vi "load_xml.vi"(8 "error in":errorcluster, 10 "child node in":refnum<k20>, 11 "Hamamatsu_C9100-13.lvclass (in)":refnum<class "Hamamatsu_C9100-13.lvclass">) -> (0 "error out":errorcluster, 2 "child node out":refnum<k20>, 3 "Hamamatsu_C9100-13.lvclass":refnum<class "Hamamatsu_C9100-13.lvclass">)   [LabVIEW 2013, in "Hamamatsu_C9100-13.lvclass"]
doc: "Loads Hamamatsu C9100-13 camera settings from xml. Expected format:\n\n<Enable>%b</Enable>\n<AnalogGain>%u</AnalogGain>\n<FrameGrabberAcquisitionRegion columns=\"left, top, right, bottom\">%u %u %u %u</FrameGrabberAcquisitionRegion>\n<ExposureTime>%f</ExposureTime>\n<EMGain>%u</EMGain>\n<TriggerPolarity>%s</TriggerPolarity>\n<ExternalTriggerMode>%s</ExternalTriggerMode>\n<ScanSpeed>%s</ScanSpeed>\n<ExternalTriggerSource>%s</ExternalTriggerSource>\n<ScanMode>%s</ScanMode>\n<SuperPixelBinning>%s</SuperPixelBinning>\n<CameraSubArrayAcquisitionRegion columns=\"left, top, width, height\">%u %u %u %u</CameraSubArrayAcquisitionRegion>\n<NumberOfImageBuffers>%u</NumberOfImageBuffers>\n<RegionsOfInterest columns=\"Left, Top, Right Bottom\">\n%s</RegionsOfInterest>\n<BackgroundRegions columns=\"Left, Top, Right Bottom\">\n%s</BackgroundRegions>\n<ShotsPerMeasurement>%u</ShotsPerMeasurement>\n<PhotoelectronScaling>%f</PhotoelectronScaling>\n\nMTL 2013 Jan 1"
uses:
  Hamamatsu_C9100-13.lvclass
  Hamamatsu_C9100-13.lvclass/Hamamatsu_C9100-13.ctl
  Experiment/Globals.vi
  <vilib>/xml/Close Reference(Node).vi
  <resource>/objmgr/DOMUserDefRef.rc
  <vilib>/xml/NI_XML.lvlib
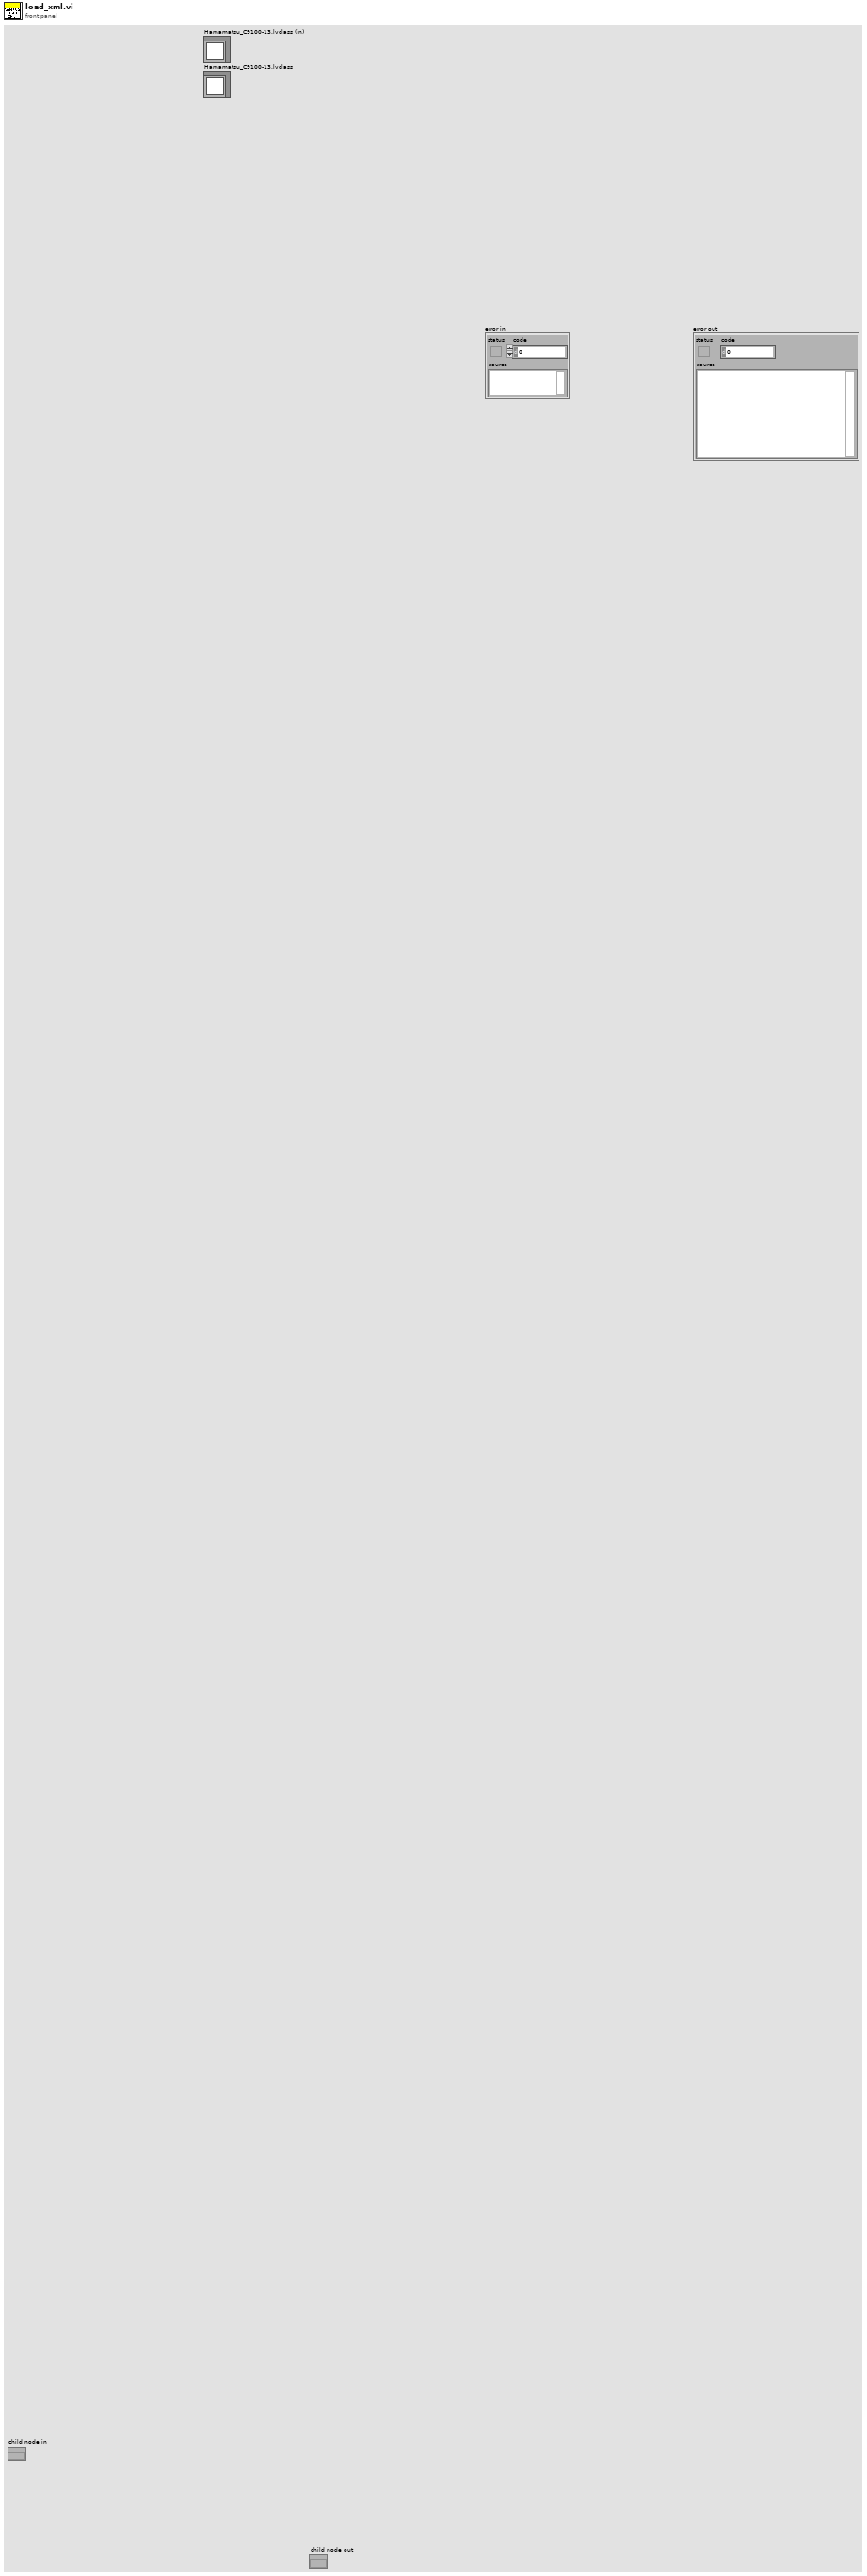
[diagram p1: front panel]
types:
  T1 = typedef "Hamamatsu_C9100-13.lvclass/camera_setup.ctl" = cluster{"Analog Gain (0-5)":u8, "Exposure Time":dbl, "EM Gain (0-255)":u8, "Trigger Polarity":string, "External Trigger Mode":string, "Scan Speed":string, "External Trigger Source":string, "Scan Mode":string, "Super Pixel Binning\n(if enabled in Scan Mode)":string, "Camera Sub-array acquisition region\n(if enabled in scan mode)":cluster{"Left":u16, "Top":u16, "Width":u16, "Height":u16}, "Use camera?":bool, "# image buffers":i32, "shots per measurement":i32, "Force images to U16":bool, "Low Light Sensitivity":string, "cooling":string, "fan":string, "Frame Grabber acquisition region":cluster{"Left":i32, "Top":i32, "Right":i32, "Bottom":i32}}
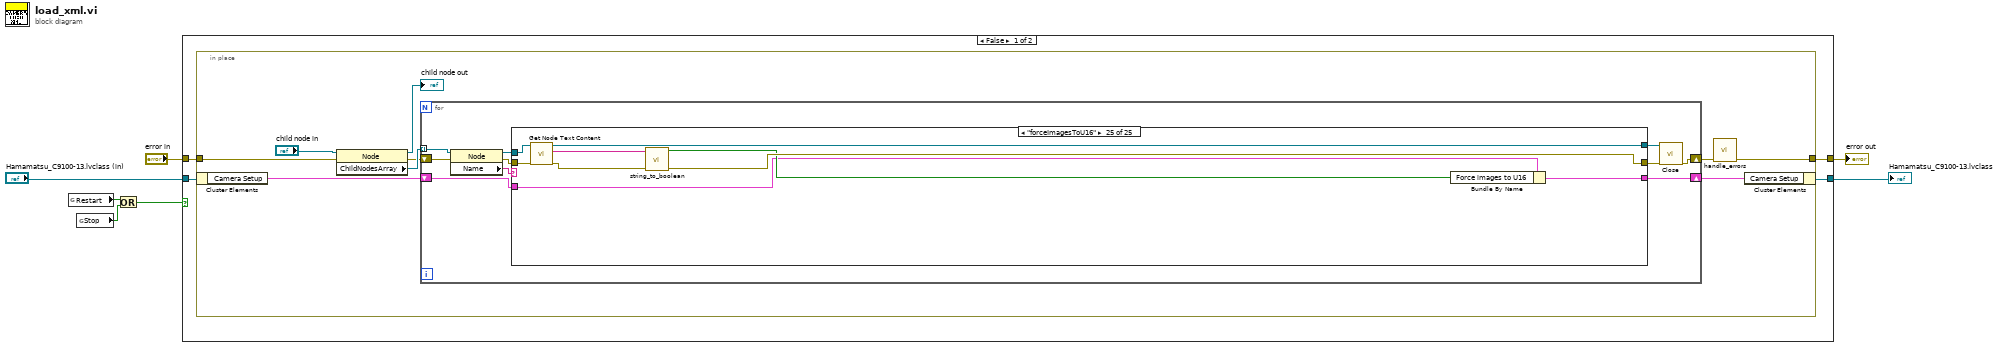
[diagram p0: block diagram]
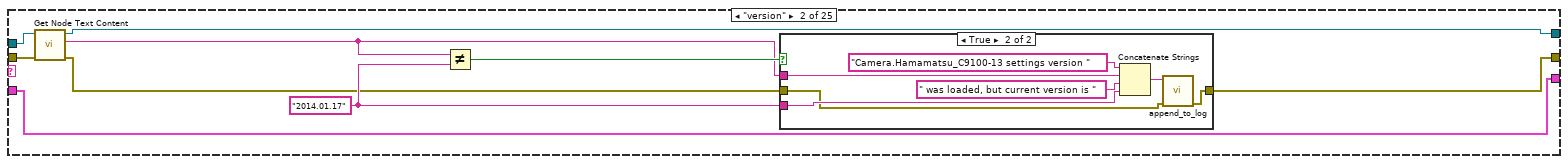
[diagram p3: hidden frame]
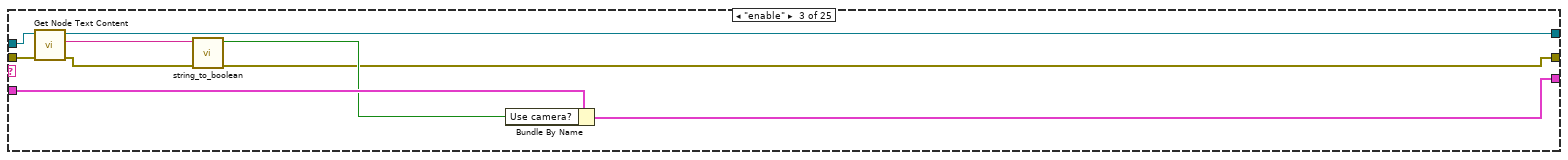
[diagram p5: hidden frame]
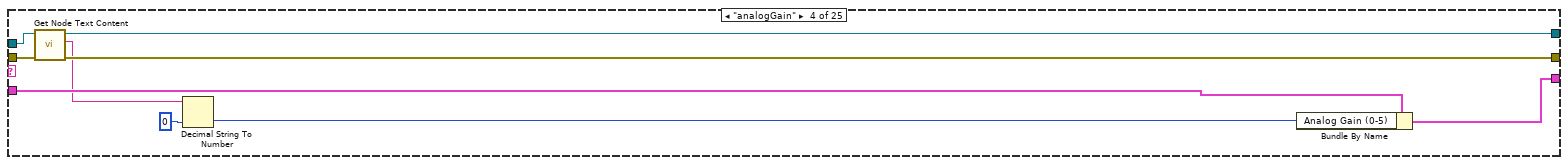
[diagram p6: hidden frame]
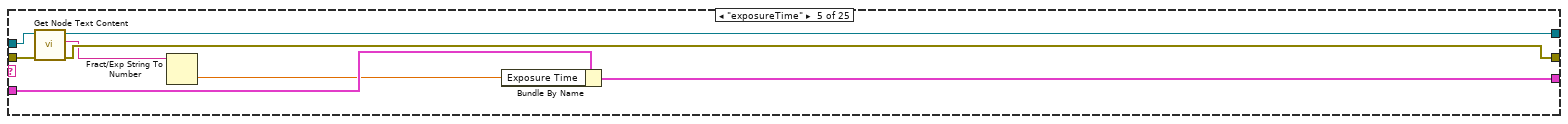
[diagram p7: hidden frame]
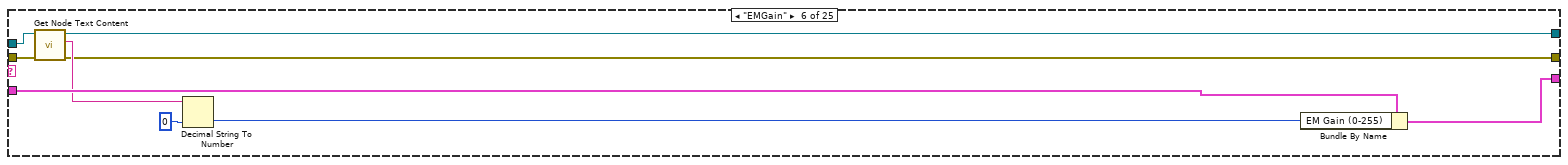
[diagram p8: hidden frame]
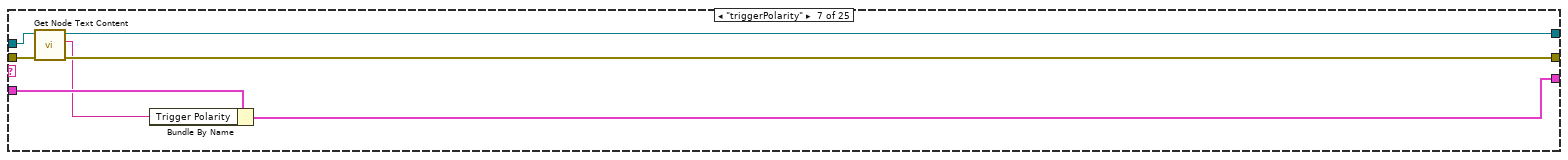
[diagram p9: hidden frame]
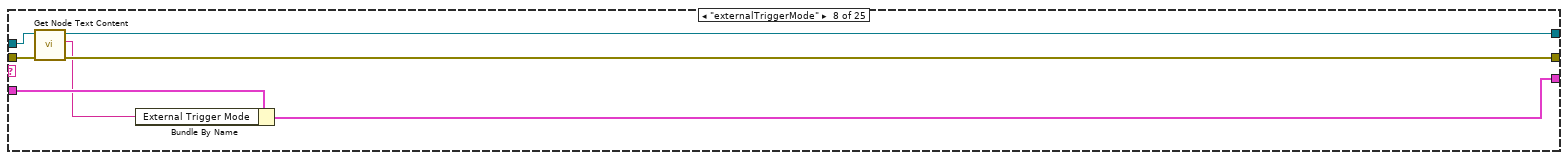
[diagram p10: hidden frame]
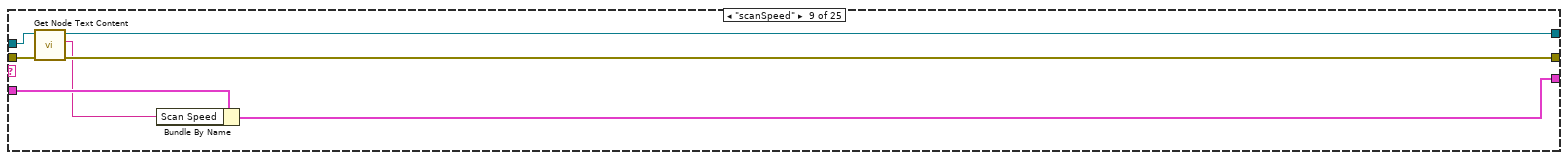
[diagram p11: hidden frame]
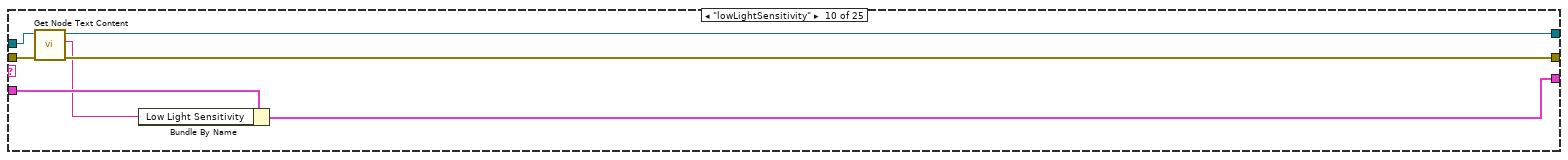
[diagram p12: hidden frame]
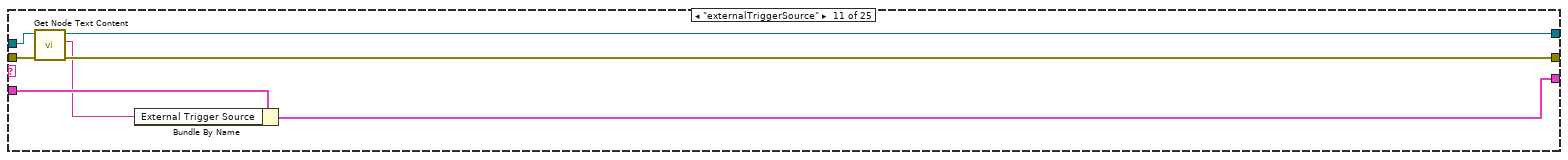
[diagram p13: hidden frame]
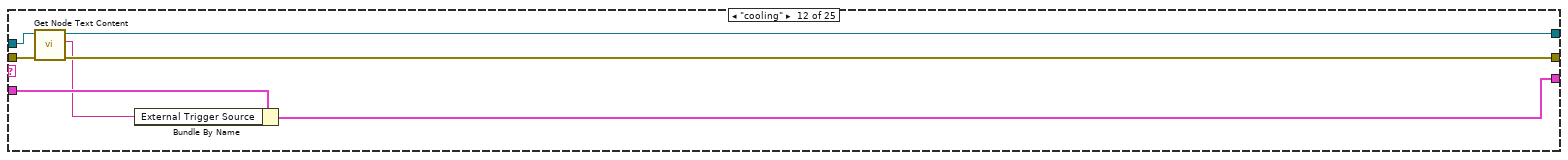
[diagram p14: hidden frame]
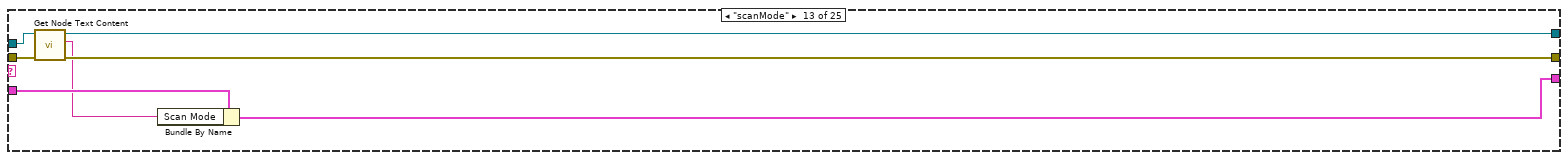
[diagram p15: hidden frame]
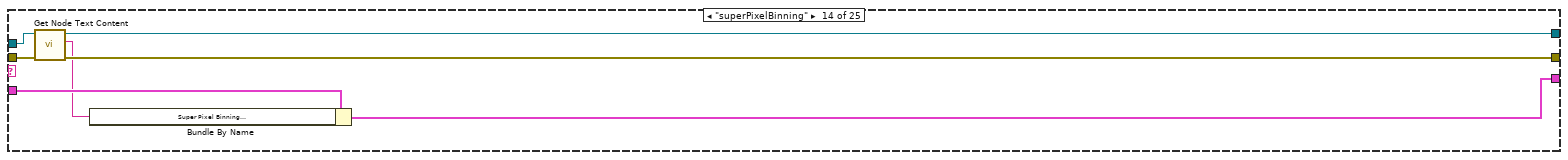
[diagram p16: hidden frame]
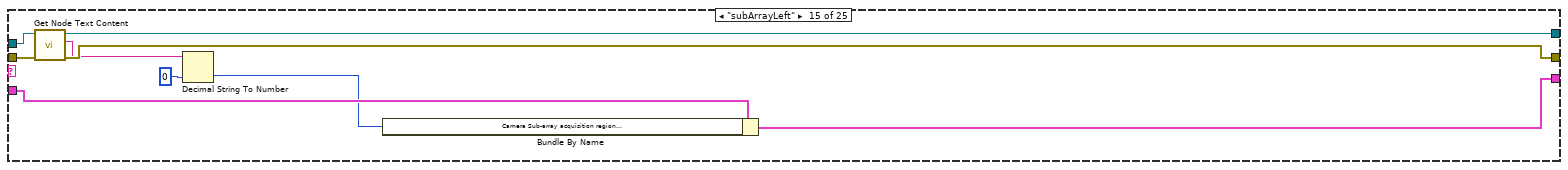
[diagram p17: hidden frame]
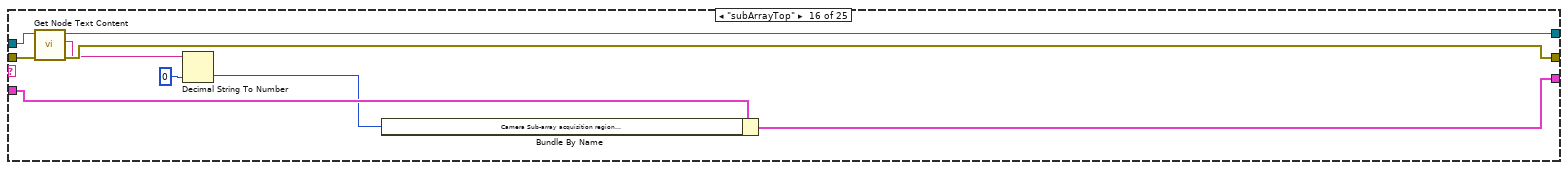
[diagram p18: hidden frame]
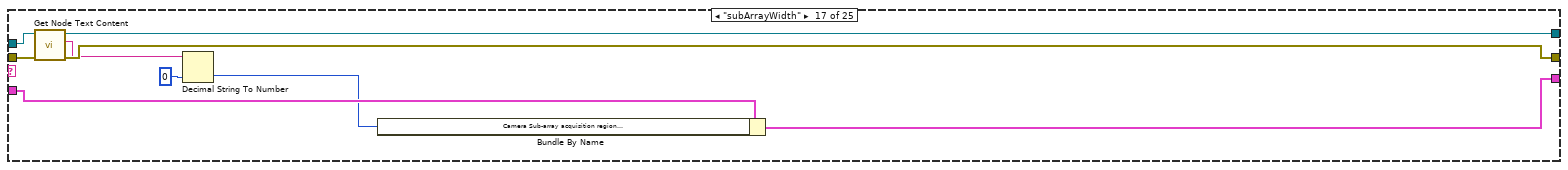
[diagram p19: hidden frame]
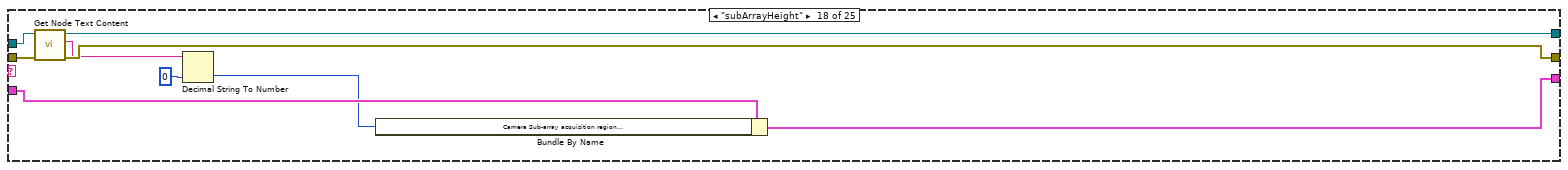
[diagram p20: hidden frame]
diagram:
  n1 = global read "Globals.vi" "Restart"() -> (w6:bool)
  n2 = global read "Globals.vi" "Stop"() -> (w5:bool)
  n3 = Or(x=w6, y=w5) -> (x .or. y?=w4:bool)
  n4 = case shown="False" w4 {
    tunnel: [w11 w242] -> w7
    tunnel: "error in" -> [w10 w242]
    tunnel: "Hamamatsu_C9100-13.lvclass (in)" -> [w9 w241]
    tunnel: [w8 w241] -> w1
    frame False {
      n5 = in-place {
        in-place-border: [w15] -> w11
        in-place-border: w10 -> [w14]
        n6 = in-place-cluster #1(w9) -> ("Camera Setup"=w12:T1)
        n7 = property class="Node"(reference="child node in", error in=w14) -> (reference out=→"child node out":refnum<k20>, error out=w18:errorcluster, "ChildNodesArray"=w20:refnum<k20>[])
        n8 = for {
          tunnel: w20 -> [w21] mode=indexing
          shift-right: [w27] -> w13
          shift-left: w12 -> [w28]
          shift-right: [w24] -> w16
          shift-left: w18 -> [w22]
          n9 = property class="Node"(reference=w21, error in=w22) -> (reference out=w29:refnum<k20>, error out=w25:errorcluster, "Name"=w30:string)
          n10 = case shown="\"forceImagesToU16\"" w30 {
            tunnel: w29 -> [w32 w37 w58 w65 w73 w84 w89 w96 w103 w110 w117 w124 w131 w138 w149 w158 w167 w176 w185 w194 w203 w212 w221 w230 w239]
            tunnel: w28 -> [w33 w36 w56 w68 w76 w82 w92 w99 w106 w113 w120 w127 w134 w141 w146 w155 w164 w173 w182 w191 w200 w209 w219 w228 w232]
            tunnel: [w33 w36 w55 w67 w75 w81 w91 w98 w105 w112 w119 w126 w133 w140 w142 w151 w160 w169 w178 w187 w196 w205 w218 w227 w237] -> w27
            tunnel: [w32 w35 w59 w66 w74 w85 w90 w97 w104 w111 w118 w125 w132 w139 w147 w156 w165 w174 w183 w192 w201 w210 w222 w231 w240] -> w26
            tunnel: w25 -> [w31 w38 w57 w64 w72 w83 w88 w95 w102 w109 w116 w123 w130 w137 w150 w159 w168 w177 w186 w195 w204 w213 w220 w229 w238]
            tunnel: [w31 w34 w51 w63 w71 w79 w87 w94 w101 w108 w115 w122 w129 w136 w148 w157 w166 w175 w184 w193 w202 w211 w216 w225 w235] -> w23
            frame "None", Default {
            }
            frame "version" {
              w40 = "2014.01.17" ("y")
              n11 = call <vilib>:"Get Node Text Content.vi"("error in (no error)"=w38, "node in"=w37) -> ("error out"=w39:errorcluster, "node text"=w41:string, "node out"=w35:refnum<k20>)  [unwired: 7 in]
              n12 = Not Equal?(x=w41, y=w40) -> (x != y?=w42:bool)
              n13 = case shown="True" w42 {
                tunnel: w41 -> [_ w49]
                tunnel: w40 -> [_ w47]
                tunnel: w39 -> [w43 w45]
                tunnel: [w43 w44] -> w34
                frame False {
                }
                frame True {
                  n14 = Concatenate Strings("Camera.Hamamatsu_C9100-13 settings version " ("string"), w49, " was loaded, but current version is " ("string"), w47) -> (w46:string)
                  n15 = call "append_to_log.vi"("error in"=w45, "string"=w46) -> ("error out"=w44:errorcluster)  [unwired: 9 in]
                }
              }
            }
            frame "enable" {
              n16 = call <vilib>:"Get Node Text Content.vi"("error in (no error)"=w57, "node in"=w58) -> ("error out"=w53:errorcluster, "node text"=w54:string, "node out"=w59:refnum<k20>)  [unwired: 7 in]
              n17 = call "string_to_boolean.vi"("error in"=w53, "string"=w54) -> ("error out"=w51:errorcluster, "boolean"=w52:bool)  [unwired: 8 in]
              n18 = Bundle By Name(cluster=w56, "Use camera?"=w52) -> (w55:T1)
            }
            frame "analogGain" {
              n19 = call <vilib>:"Get Node Text Content.vi"("error in (no error)"=w64, "node in"=w65) -> ("error out"=w63:errorcluster, "node text"=w62:string, "node out"=w66:refnum<k20>)  [unwired: 7 in]
              n20 = Decimal String To Number(string=w62, default (0L)=u8 0 ("Analog Gain (0-5)")) -> (number=w60:u8)  [unwired: 1 in, 1 out]
              n21 = Bundle By Name(cluster=w68, "Analog Gain (0-5)"=w60) -> (w67:T1)
            }
            frame "exposureTime" {
              n22 = call <vilib>:"Get Node Text Content.vi"("error in (no error)"=w72, "node in"=w73) -> ("error out"=w71:errorcluster, "node text"=w70:string, "node out"=w74:refnum<k20>)  [unwired: 7 in]
              n23 = Fract/Exp String To Number(string=w70) -> (number=w69:dbl)  [unwired: 3 in, 1 out]
              n24 = Bundle By Name(cluster=w76, "Exposure Time"=w69) -> (w75:T1)
            }
            frame "EMGain" {
              n25 = call <vilib>:"Get Node Text Content.vi"("error in (no error)"=w83, "node in"=w84) -> ("error out"=w79:errorcluster, "node text"=w80:string, "node out"=w85:refnum<k20>)  [unwired: 7 in]
              n26 = Decimal String To Number(string=w80, default (0L)=u8 0 ("EM Gain (0-255)")) -> (number=w77:u8)  [unwired: 1 in, 1 out]
              n27 = Bundle By Name(cluster=w82, "EM Gain (0-255)"=w77) -> (w81:T1)
            }
            frame "triggerPolarity" {
              n28 = call <vilib>:"Get Node Text Content.vi"("error in (no error)"=w88, "node in"=w89) -> ("error out"=w87:errorcluster, "node text"=w86:string, "node out"=w90:refnum<k20>)  [unwired: 7 in]
              n29 = Bundle By Name(cluster=w92, "Trigger Polarity"=w86) -> (w91:T1)
            }
            frame "externalTriggerMode" {
              n30 = call <vilib>:"Get Node Text Content.vi"("error in (no error)"=w95, "node in"=w96) -> ("error out"=w94:errorcluster, "node text"=w93:string, "node out"=w97:refnum<k20>)  [unwired: 7 in]
              n31 = Bundle By Name(cluster=w99, "External Trigger Mode"=w93) -> (w98:T1)
            }
            frame "scanSpeed" {
              n32 = call <vilib>:"Get Node Text Content.vi"("error in (no error)"=w102, "node in"=w103) -> ("error out"=w101:errorcluster, "node text"=w100:string, "node out"=w104:refnum<k20>)  [unwired: 7 in]
              n33 = Bundle By Name(cluster=w106, "Scan Speed"=w100) -> (w105:T1)
            }
            frame "lowLightSensitivity" {
              n34 = call <vilib>:"Get Node Text Content.vi"("error in (no error)"=w109, "node in"=w110) -> ("error out"=w108:errorcluster, "node text"=w107:string, "node out"=w111:refnum<k20>)  [unwired: 7 in]
              n35 = Bundle By Name(cluster=w113, "Low Light Sensitivity"=w107) -> (w112:T1)
            }
            frame "externalTriggerSource" {
              n36 = call <vilib>:"Get Node Text Content.vi"("error in (no error)"=w116, "node in"=w117) -> ("error out"=w115:errorcluster, "node text"=w114:string, "node out"=w118:refnum<k20>)  [unwired: 7 in]
              n37 = Bundle By Name(cluster=w120, "External Trigger Source"=w114) -> (w119:T1)
            }
            frame "cooling" {
              n38 = call <vilib>:"Get Node Text Content.vi"("error in (no error)"=w123, "node in"=w124) -> ("error out"=w122:errorcluster, "node text"=w121:string, "node out"=w125:refnum<k20>)  [unwired: 7 in]
              n39 = Bundle By Name(cluster=w127, "External Trigger Source"=w121) -> (w126:T1)
            }
            frame "scanMode" {
              n40 = call <vilib>:"Get Node Text Content.vi"("error in (no error)"=w130, "node in"=w131) -> ("error out"=w129:errorcluster, "node text"=w128:string, "node out"=w132:refnum<k20>)  [unwired: 7 in]
              n41 = Bundle By Name(cluster=w134, "Scan Mode"=w128) -> (w133:T1)
            }
            frame "superPixelBinning" {
              n42 = call <vilib>:"Get Node Text Content.vi"("error in (no error)"=w137, "node in"=w138) -> ("error out"=w136:errorcluster, "node text"=w135:string, "node out"=w139:refnum<k20>)  [unwired: 7 in]
              n43 = Bundle By Name(cluster=w141, "Super Pixel Binning\n(if enabled in Scan Mode)"=w135) -> (w140:T1)
            }
            frame "subArrayLeft" {
              n44 = call <vilib>:"Get Node Text Content.vi"("error in (no error)"=w150, "node in"=w149) -> ("error out"=w148:errorcluster, "node text"=w144:string, "node out"=w147:refnum<k20>)  [unwired: 7 in]
              n45 = Decimal String To Number(string=w144, default (0L)=u16 0 ("EM Gain (0-255)")) -> (number=w143:u16)  [unwired: 1 in, 1 out]
              n46 = Bundle By Name(cluster=w146, "Camera Sub-array acquisition region\n(if enabled in scan mode).Left"=w143) -> (w142:T1)
            }
            frame "subArrayTop" {
              n47 = call <vilib>:"Get Node Text Content.vi"("error in (no error)"=w159, "node in"=w158) -> ("error out"=w157:errorcluster, "node text"=w153:string, "node out"=w156:refnum<k20>)  [unwired: 7 in]
              n48 = Decimal String To Number(string=w153, default (0L)=u16 0 ("EM Gain (0-255)")) -> (number=w152:u16)  [unwired: 1 in, 1 out]
              n49 = Bundle By Name(cluster=w155, "Camera Sub-array acquisition region\n(if enabled in scan mode).Top"=w152) -> (w151:T1)
            }
            frame "subArrayWidth" {
              n50 = call <vilib>:"Get Node Text Content.vi"("error in (no error)"=w168, "node in"=w167) -> ("error out"=w166:errorcluster, "node text"=w162:string, "node out"=w165:refnum<k20>)  [unwired: 7 in]
              n51 = Decimal String To Number(string=w162, default (0L)=u16 0 ("EM Gain (0-255)")) -> (number=w161:u16)  [unwired: 1 in, 1 out]
              n52 = Bundle By Name(cluster=w164, "Camera Sub-array acquisition region\n(if enabled in scan mode).Width"=w161) -> (w160:T1)
            }
            frame "subArrayHeight" {
              n53 = call <vilib>:"Get Node Text Content.vi"("error in (no error)"=w177, "node in"=w176) -> ("error out"=w175:errorcluster, "node text"=w171:string, "node out"=w174:refnum<k20>)  [unwired: 7 in]
              n54 = Decimal String To Number(string=w171, default (0L)=u16 0 ("EM Gain (0-255)")) -> (number=w170:u16)  [unwired: 1 in, 1 out]
              n55 = Bundle By Name(cluster=w173, "Camera Sub-array acquisition region\n(if enabled in scan mode).Height"=w170) -> (w169:T1)
            }
            frame "frameGrabberAcquisitionRegionLeft" {
              n56 = call <vilib>:"Get Node Text Content.vi"("error in (no error)"=w186, "node in"=w185) -> ("error out"=w184:errorcluster, "node text"=w180:string, "node out"=w183:refnum<k20>)  [unwired: 7 in]
              n57 = Decimal String To Number(string=w180, default (0L)=0 ("EM Gain (0-255)")) -> (number=w179:i32)  [unwired: 1 in, 1 out]
              n58 = Bundle By Name(cluster=w182, "Frame Grabber acquisition region.Left"=w179) -> (w178:T1)
            }
            frame "frameGrabberAcquisitionRegionTop" {
              n59 = call <vilib>:"Get Node Text Content.vi"("error in (no error)"=w195, "node in"=w194) -> ("error out"=w193:errorcluster, "node text"=w189:string, "node out"=w192:refnum<k20>)  [unwired: 7 in]
              n60 = Decimal String To Number(string=w189, default (0L)=0 ("EM Gain (0-255)")) -> (number=w188:i32)  [unwired: 1 in, 1 out]
              n61 = Bundle By Name(cluster=w191, "Frame Grabber acquisition region.Top"=w188) -> (w187:T1)
            }
            frame "frameGrabberAcquisitionRegionRight" {
              n62 = call <vilib>:"Get Node Text Content.vi"("error in (no error)"=w204, "node in"=w203) -> ("error out"=w202:errorcluster, "node text"=w198:string, "node out"=w201:refnum<k20>)  [unwired: 7 in]
              n63 = Decimal String To Number(string=w198, default (0L)=0 ("EM Gain (0-255)")) -> (number=w197:i32)  [unwired: 1 in, 1 out]
              n64 = Bundle By Name(cluster=w200, "Frame Grabber acquisition region.Right"=w197) -> (w196:T1)
            }
            frame "frameGrabberAcquisitionRegionBottom" {
              n65 = call <vilib>:"Get Node Text Content.vi"("error in (no error)"=w213, "node in"=w212) -> ("error out"=w211:errorcluster, "node text"=w207:string, "node out"=w210:refnum<k20>)  [unwired: 7 in]
              n66 = Decimal String To Number(string=w207, default (0L)=0 ("EM Gain (0-255)")) -> (number=w206:i32)  [unwired: 1 in, 1 out]
              n67 = Bundle By Name(cluster=w209, "Frame Grabber acquisition region.Bottom"=w206) -> (w205:T1)
            }
            frame "NumberOfImageBuffers" {
              n68 = call <vilib>:"Get Node Text Content.vi"("error in (no error)"=w220, "node in"=w221) -> ("error out"=w216:errorcluster, "node text"=w217:string, "node out"=w222:refnum<k20>)  [unwired: 7 in]
              n69 = Decimal String To Number(string=w217, default (0L)=0 ("EM Gain (0-255)")) -> (number=w214:i32)  [unwired: 1 in, 1 out]
              n70 = Bundle By Name(cluster=w219, "# image buffers"=w214) -> (w218:T1)
            }
            frame "ShotsPerMeasurement" {
              n71 = call <vilib>:"Get Node Text Content.vi"("error in (no error)"=w229, "node in"=w230) -> ("error out"=w225:errorcluster, "node text"=w226:string, "node out"=w231:refnum<k20>)  [unwired: 7 in]
              n72 = Decimal String To Number(string=w226, default (0L)=0 ("EM Gain (0-255)")) -> (number=w223:i32)  [unwired: 1 in, 1 out]
              n73 = Bundle By Name(cluster=w228, "shots per measurement"=w223) -> (w227:T1)
            }
            frame "forceImagesToU16" {
              n74 = call <vilib>:"Get Node Text Content.vi"("error in (no error)"=w238, "node in"=w239) -> ("error out"=w236:errorcluster, "node text"=w234:string, "node out"=w240:refnum<k20>)  [unwired: 7 in]
              n75 = call "string_to_boolean.vi"("error in"=w236, "string"=w234) -> ("error out"=w235:errorcluster, "boolean"=w233:bool)  [unwired: 8 in]
              n76 = Bundle By Name(cluster=w232, "Force images to U16"=w233) -> (w237:T1)
            }
          }
          n77 = call-poly <vilib>:"Close.vi"("error in (no error)"=w23, "node"=w26) -> ("error out"=w24:errorcluster)  [unwired: 7 in]
        }
        n78 = call "handle_errors.vi"("error in (no error)"=w16) -> ("error out"=w15:errorcluster)  [unwired: 10 in]
        n79 = in-place-cluster #1("Camera Setup"=w13) -> (w8:refnum<class "Hamamatsu_C9100-13.lvclass">)
      }
    }
    frame True {
    }
  }
  "error out" <- w7
  "Hamamatsu_C9100-13.lvclass" <- w1
